vi "Rohde & Schwarz VNA Set Learn String.vi"(7 "Rohde & Schwarz VNA":T1, 8 "error in (no error)":errorcluster, 10 "Learn String":string, 11 "VISA Resource Name":refnum<visa-resource-name>) -> (0 "error out":errorcluster {"code" format="%.0x"}, 3 "dup VISA Resource Name":refnum<visa-resource-name>)   [LabVIEW 2011]
uses:
  TypeDefs/Rohde & Schwarz VNA Instrument Info.ctl
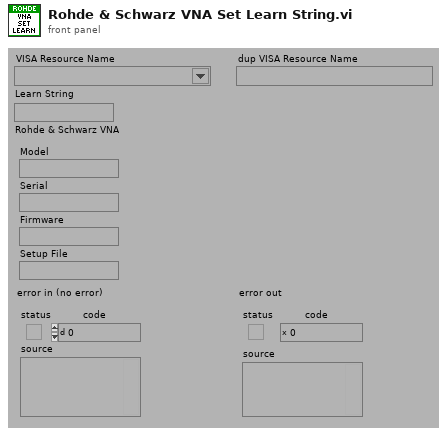
[diagram p1: front panel]
types:
  T1 = typedef "Rohde & Schwarz VNA Instrument Info.ctl" = cluster{"Model":string, "Serial":string, "Firmware":string, "Setup File":string}
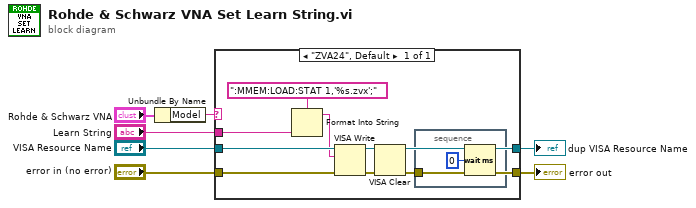
[diagram p0: block diagram]
diagram:
  n1 = Unbundle By Name("Rohde & Schwarz VNA") -> ("Model"=w2:string)
  n2 = case shown="\"ZVA24\", Default" w2 {
    tunnel: [w9] -> w7
    tunnel: "error in (no error)" -> [w16]
    tunnel: "VISA Resource Name" -> [w15]
    tunnel: [w10] -> w4
    tunnel: "Learn String" -> [w8]
    frame "ZVA24", Default {
      n3 = Format Into String(format string=":MMEM:LOAD:STAT 1,'%s.zvx';", w8) -> (resulting string=w13:string)  [unwired: 2 in, 1 out]
      n4 = VISA Write(VISA resource name=w15, write buffer=w13, error in (no error)=w16) -> (VISA resource name out=w11:refnum<visa-resource-name>, error out=w12:errorcluster)  [unwired: 1 out]
      n5 = VISA Clear(VISA resource name=w11, error in (no error)=w12) -> (VISA resource name out=w10:refnum<visa-resource-name>, error out=w9:errorcluster)
      n6 = stacked-sequence {
        tunnel: w9 -> [_]
        frame #0 {
          n7 = Wait (ms)(milliseconds to wait=u32 0) -> ()  [unwired: 1 out]
        }
      }
    }
  }
  "error out" <- w7
  "dup VISA Resource Name" <- w4
